vi "Create User Event - EHL Stop.vi"(8 "error in":errorcluster) -> (0 "error out":errorcluster, 3 "User Event":refnum<user-event>)   [LabVIEW 2016, in "User Event - EHL Stop.lvlib"]
doc: "Creates a boolean user event that stops the event loop from the message handling loop"
uses:
  User Event - EHL Stop.lvlib
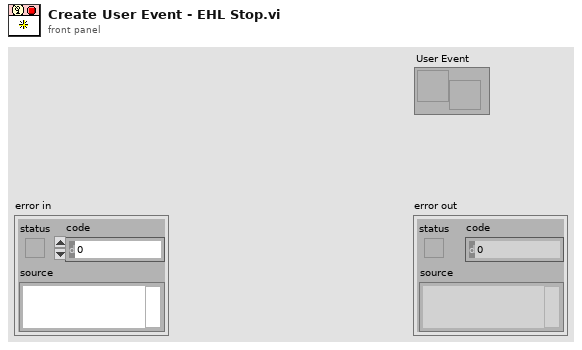
[diagram p1: front panel]
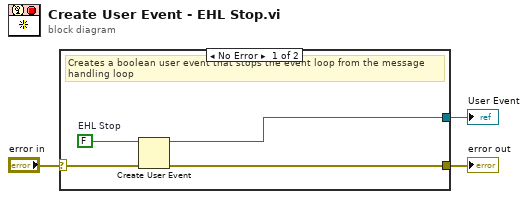
[diagram p0: block diagram]
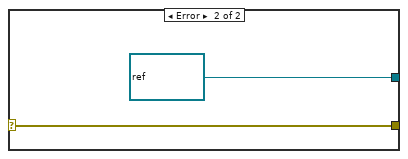
[diagram p2: hidden frame]
diagram:
  n1 = case shown="No Error" "error in" {
    selector: "error in" -> [w4 w9]
    tunnel: [w7 refnum<user-event> refnum ("EHL Stop")] -> w3
    tunnel: [w5 w9] -> w2
    frame No Error {
      w6 = FALSE  # EHL Stop
      # "Creates a boolean user event that stops the event loop from the message handling loop"
      n2 = Create User Event(user event datatype=w6, error in=w4) -> (user event=w7:refnum<user-event>, error out=w5:errorcluster)
    }
    frame Error {
    }
  }
  "User Event" <- w3
  "error out" <- w2
